vi "Fetch Waveform_Mod.vi"(0 "VISA resource name":refnum<visa-resource-name>, 1 "First point (0: First point)":i32, 3 "Number of points (0: All points)":i32, 5 "Source (0: Channel 1)":u16(ring) items=["Channel 1", "Channel 2", "Channel 3", "Channel 4", "Memory 1", "Memory 2", "Memory 3", "Memory 4", "Function 1", "Function 2", "Function 3", "Function 4", "Function 5", "Function 6", "Function 7", "Function 8", "Other"], 9 "Timeout (10000 ms)":u32=10000, 11 "error in (no error)":errorcluster, 12 "Segment number (0: All segment)":i16, 14 "Sparsing (0: Every point)":i32) -> (4 "VISA resource name out":refnum<visa-resource-name>, 6 "Waveform Graph":waveform(dbl)(graph), 8 "Nom_Bits":i16, 10 "Raw Data":i16[](array[numeric]), 13 "Horizontal Offset":dbl, 15 "error out":errorcluster)   [LabVIEW 2022 SP3]
doc: "Returns the waveform the oscilloscope acquired for the specified channel. The waveform is from an acquisition that you initiate prior to calling this VI.\n\nYou use the Initiate VI to start an acquisition on the channels that you enable with the <B>Configure Channel</B> VI. The oscilloscope acquires waveforms for the enabled channels concurrently. You must call this VI separately for each enabled channel to obtain the waveforms.\n\nYou can call the <B>lcwave Read Single Waveform</B> VI or <B>lcwave Read Multiple Waveforms</B> VI instead of using low level VIs.\n\n<B>Note</B> This VI does not check the instrument status. Typically, you call this VI only in a sequence of calls to other low-level instrument driver VIs. The sequence performs one operation. You use the low-level VIs to optimize one or more aspects of interaction with the instrument."
uses:
  <instrlib>/LeCroy Wave Series/LeCroy Wave Series.lvlib
panel:
  in  "Custom Source ID":string
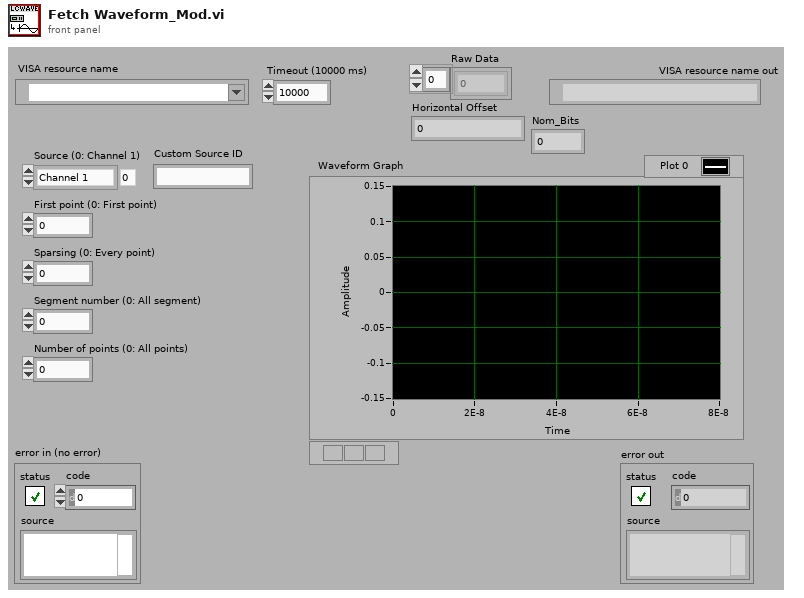
[diagram p1: front panel]
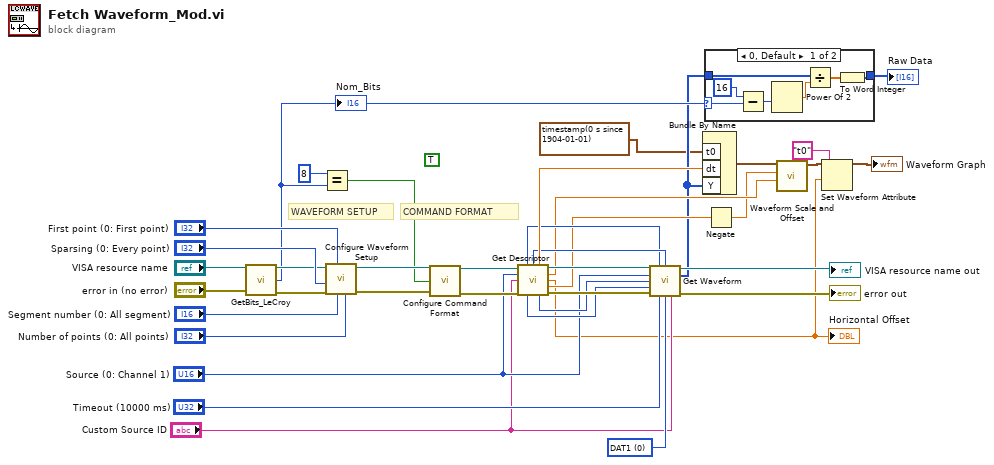
[diagram p0: block diagram]
diagram:
  (unwired) TRUE ("Command format (T: Byte)")
  w28 = u16 0 items=["DAT1", "DAT2"] ("Array (1: DAT1)")
  # "WAVEFORM SETUP"
  # "COMMAND FORMAT"
  n1 = call "GetBits_LeCroy.vi"("VISA resource name"="VISA resource name", "error in (no error)"="error in (no error)") -> ("VISA resource name out"=w11:refnum<visa-resource-name>, "Nom_Bits"=w7:i16, "error out"=w12:errorcluster)  [unwired: 11 in]
  "Nom_Bits" <- w7
  n2 = Equal?(x=8, y=w7) -> (x = y?=w8:bool)
  n3 = call <instrlib>:"Configure Waveform Setup.vi"("Number of points (0: All points)"="Number of points (0: All points)", "Segment number (0: All segment)"="Segment number (0: All segment)", "First point (0: First point)"="First point (0: First point)", "error in (no error)"=w12, "Sparsing (0: Every point)"="Sparsing (0: Every point)", "VISA resource name"=w11) -> ("error out"=w33:errorcluster, "VISA resource name out"=w34:refnum<visa-resource-name>)  [unwired: 4 in]
  n4 = call <instrlib>:"Configure Command Format.vi"("VISA resource name"=w34, "Command format (T: Byte)"=w8, "error in (no error)"=w33) -> ("VISA resource name out"=w26:refnum<visa-resource-name>, "error out"=w25:errorcluster)  [unwired: 11 in]
  n5 = call <instrlib>:"Get Descriptor.vi"("VISA resource name"=w26, "Source (0: Channel 1)"="Source (0: Channel 1)", "Custom Source ID"="Custom Source ID", "error in (no error)"=w25) -> ("First Valid Point"=w22:i32, "Last Valid Point"=w23:i32, "Horizontal interval"=w29:sgl, "VISA resource name out"=w39:refnum<visa-resource-name>, "Vertical gain"=w19:sgl, "Horizontal Offset"=w1:dbl, "Vertical offset"=w18:sgl, "Number Of Data Points"=w27:i32, "Command type"=w35:i16, "error out"=w38:errorcluster)  [unwired: 1 in, 1 out]
  "Horizontal Offset" <- w1
  n6 = call <instrlib>:"Get Waveform.vi"("VISA resource name"=w39, "First Valid Point"=w22, "Last Valid Point"=w23, "Source (0: Channel 1)"="Source (0: Channel 1)", "Command type (0: byte)"=w35, "Number Of Data Points (10000)"=w27, "error in (no error)"=w38, "Timeout (10000 ms)"="Timeout (10000 ms)", "Array (0: DAT1)"=w28, "Custom Source ID"="Custom Source ID") -> ("VISA resource name out"=→"VISA resource name out":refnum<visa-resource-name>, "Waveform Graph"=w6:i16[], "error out"=→"error out":errorcluster)  [unwired: 3 in]
  n7 = Bundle By Name ("Build Waveform")("t0"=timestamp(0 s since 1904-01-01), "dt"=w29, "Y"=w6) -> (w21:waveform(i16))  [unwired: 1 in]
  n8 = case shown="0, Default" w7 {
    selector: w7 -> [w44 _]
    tunnel: w6 -> [w45 w47]
    tunnel: [w40 w47] -> w5
    frame 0, Default {
      n9 = Subtract(x=16, y=w44) -> (x-y=w42:i32)
      n10 = Power Of 2(x=w42) -> (2^x=w41:dbl)
      n11 = Divide(x=w45, y=w41) -> (x/y=w46:dbl[])
      n12 = To Word Integer(number=w46) -> (16bit integer=w40:i16[])
    }
    frame 8 {
    }
  }
  "Raw Data" <- w5
  n13 = Negate(x=w18) -> (-x=w17:sgl)
  n14 = call <vilib>:"Waveform Scale and Offset.vi"("scale"=w19, "offset"=w17, "waveform in"=w21) -> ("waveform out"=w20:waveform(dbl))  [unwired: 7 in, 1 out]
  n15 = Set Waveform Attribute(5:w1, 6:"t0" ("name"), 7:w20) -> (3:→"Waveform Graph":waveform(dbl))  [unwired: 1 in, 2 out]
